vi "DAC V vs freq sweep.vi"() -> ()   [LabVIEW 2012]
uses:
  <vilib>/Analysis/1siggen.llb/Ramp Pattern by Samples.vi
  <vilib>/Utility/file.llb/Write To Spreadsheet File (DBL).vi
  <vilib>/Analysis/NI_AALBase.lvlib
panel:
  in  "file path (dialog if empty)":path
  in  "resolution (1 Hz:1)":i32(ring)=1 items=["0.1 Hz", "1 Hz", "10 Hz", "100 Hz", "1 KHz", "10 KHz", "100 KHz", "1 MHz", "10 MHz", "100 MHz", "1 GHz"]
  in  "band (1-26.5 GHz:20)":i32(ring)=2
  in  "GPIB Address":string="19"
  in  "start":dbl format="%0.2f"
  in  "end":dbl=1.0 format="%0.2f"
  in  "samples":i32=128
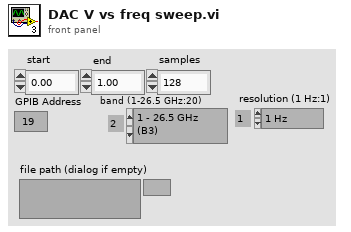
[diagram p1: front panel]
types:
  T1 = cluster{"source lock":bool, "lock frequency (Hz)":ext, "coarse tune":bool}
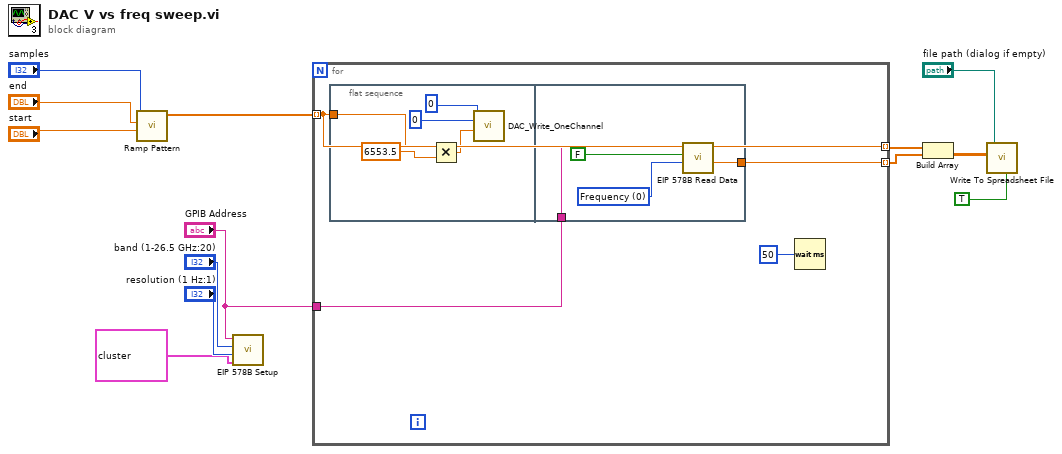
[diagram p0: block diagram]
diagram:
  n1 = call-poly <vilib>:"Ramp Pattern.vi"("start"="start", "end"="end", "samples"="samples") -> ("Ramp Pattern"=w10:dbl[])  [unwired: 7 in, 1 out]
  n2 = call "EIP 578B Setup.vi"("GPIB Address"="GPIB Address", "band (1-26.5 GHz:20)"="band (1-26.5 GHz:20)", "resolution (1 Hz:1)"="resolution (1 Hz:1)", "source locking"=T1 {"source lock"=FALSE, "lock frequency (Hz)"=1000000000.0, "coarse tune"=TRUE}) -> ()  [unwired: 2 in, 2 out]
  n3 = for {
    tunnel: w10 -> [w15] mode=indexing
    tunnel: "GPIB Address" -> [w17]
    tunnel: [w16] -> w4 mode=indexing
    tunnel: [w15] -> w5 mode=indexing
    n4 = flat-sequence {
      tunnel: w15 -> [w18]
      tunnel: w17 -> [w24]
      tunnel: [w23] -> w16
      frame #0 {
        n5 = Multiply(x=w18, y=6553.5) -> (x*y=w21:dbl)
        n6 = call "DAC_Write_OneChannel.vi"("Value"=w21, "Channel"=u16 0, "DeviceIndex"=u64 0) -> ()  [unwired: 7 in, 2 out]
      }
      frame #1 {
        w26 = 0 items=["Frequency", "Power", "Both"] ("output mode (freq:0)")
        n7 = call "EIP 578B Read Data.vi"("output mode (freq:0)"=w26, "fast (T=active)"=FALSE, "GPIB"=w24) -> ("frequency (Hz)"=w23:ext)  [unwired: 1 in, 3 out]
      }
    }
    n8 = Wait (ms)(milliseconds to wait=u32 50) -> ()  [unwired: 1 out]
  }
  n9 = Build Array(w5, w4) -> (w3:ext[][])
  n10 = call-poly <vilib>:"Write To Spreadsheet File.vi"("transpose? (no:F)"=TRUE, "2D data"=w3, "file path (dialog if empty)"="file path (dialog if empty)") -> ()  [unwired: 5 in, 1 out]
